vi "Apply Delay.vi"(6 "Delay?":bool, 8 "Levels":u8, 9 "Element in":fxp<+/-,8,8>) -> (1 "Element out":fxp<+/-,8,8>)   [LabVIEW 2015]
doc: "Attenuates the delayed signal and adds it to the input signal to achieve the desired echo effect."
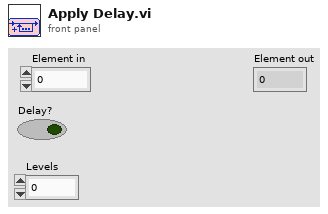
[diagram p1: front panel]
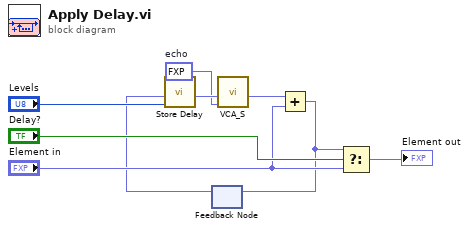
[diagram p0: block diagram]
diagram:
  w1 = fxp<+,8,0> 0.75  # echo
  n1 = feedback #1() -> (w2:fxp<+/-,8,8>)  [unwired: 1 in]
  n2 = call "Store Delay.vi"("Levels"="Levels", "Data In"=w2) -> ("Data Out"=w5:fxp<+/-,8,8>)  [unwired: 9 in]
  n3 = call "VCA_S.vi"("Amount"=w1, "Sample In"=w5) -> ("Sample Out"=w4:fxp<+/-,8,8>)  [unwired: 9 in]
  n4 = Add(x=w4, y="Element in") -> (x+y=w3:fxp<+/-,8,8>)
  n5 = feedback-in #1(w3) -> ()
  n6 = Select(t=w3, s="Delay?", f="Element in") -> (s? t:f=→"Element out":fxp<+/-,8,8>)
